vi "start ROI set-CCD1.vi"(0 "Rectangle big CCD1":T3 {"Rotation" format="%.2f"; "Left" scale=0.0..1024.0; "Right" scale=0.0..1024.0}, 1 "Rectangle small CCD1":T3 {"Rotation" format="%.2f"; "Left" scale=0.0..1024.0; "Right" scale=0.0..1024.0}, 2 "Line":T2 {"Start X" scale=0.0..1024.0; "End X" scale=0.0..1024.0}, 3 "Rectangle top CCD1":T3 {"Rotation" format="%.2f"; "Left" scale=0.0..1024.0; "Right" scale=0.0..1024.0}) -> (7 "ROI Descriptor (big)":T1={"Global Rectangle"=[1279, 916, 1775, 986], "Contours"=[{"ID"=enum."External", "Type"=12, "Coordinates"=[1280, 918, 1774, 984, 180289]}]} {"Contours"."Type" items=["No Selection", "Point", "Line", "Rectangle", "Oval", "Polygon", "Freehand Region", "Annulus", "Unused2", "Unused3", "Broken Line", "Freehand Line", "Rotated Rectangle"]}, 8 "ROI Descriptor (Small)":T1={"Global Rectangle"=[1279, 916, 1775, 986], "Contours"=[{"ID"=enum."External", "Type"=12, "Coordinates"=[1280, 918, 1774, 984, 180289]}]} {"Contours"."Type" items=["No Selection", "Point", "Line", "Rectangle", "Oval", "Polygon", "Freehand Region", "Annulus", "Unused2", "Unused3", "Broken Line", "Freehand Line", "Rotated Rectangle"]}, 9 "ROI Descriptor top":T1={"Global Rectangle"=[1279, 916, 1775, 986], "Contours"=[{"ID"=enum."External", "Type"=12, "Coordinates"=[1280, 918, 1774, 984, 180289]}]} {"Contours"."Type" items=["No Selection", "Point", "Line", "Rectangle", "Oval", "Polygon", "Freehand Region", "Annulus", "Unused2", "Unused3", "Broken Line", "Freehand Line", "Rotated Rectangle"]}, 10 "ROI Descriptor LINE":T1={"Global Rectangle"=[666, 165, 1207, 166], "Contours"=[{"ID"=enum."External", "Type"=2, "Coordinates"=[666, 165, 1206, 165]}]} {"Contours"."Type" items=["No Selection", "Point", "Line", "Rectangle", "Oval", "Polygon", "Freehand Region", "Annulus", "Unused2", "Unused3", "Broken Line", "Freehand Line", "Rotated Rectangle"]})   [LabVIEW 2017]
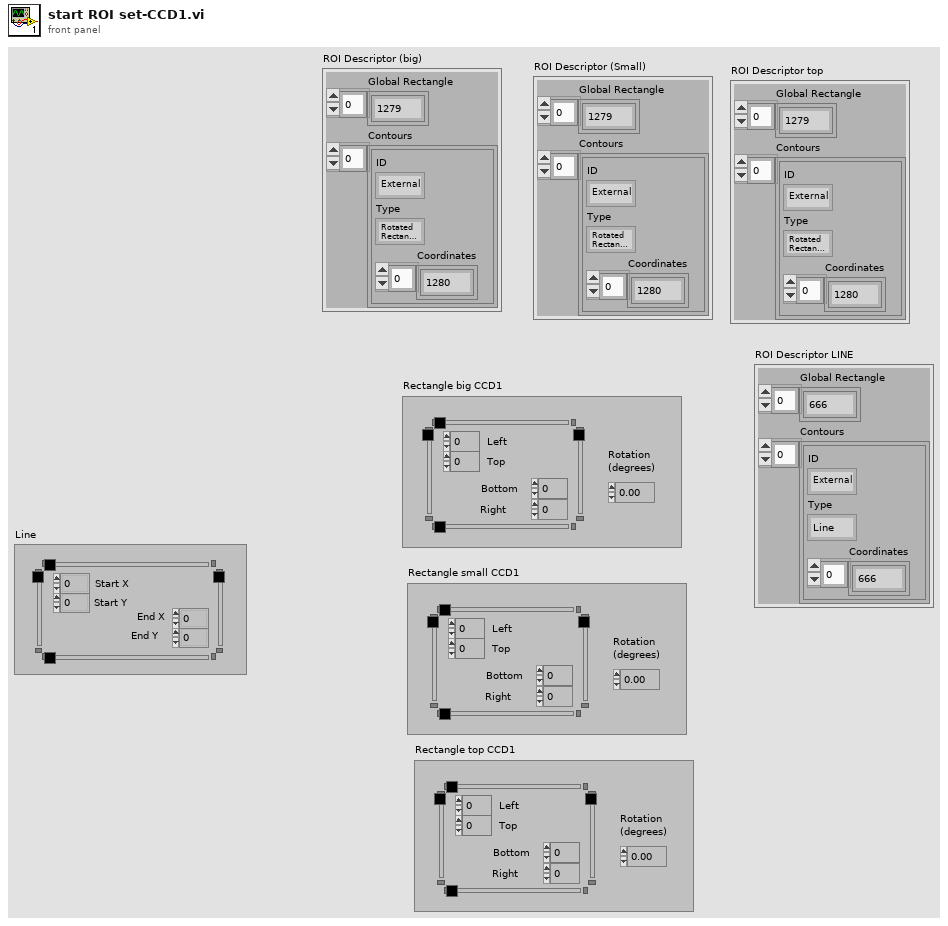
[diagram p1: front panel]
types:
  T1 = cluster{"Global Rectangle":i32[], "Contours":cluster{"ID":enum32{"External", "Internal"}, "Type":u32, "Coordinates":i32[]}[]}
  T2 = typedef "IMAQ Line" = cluster{"Start X":i32, "Start Y":i32, "End X":i32, "End Y":i32}
  T3 = typedef "IMAQ Rectangle" = cluster{"Left":i32, "Top":i32, "Right":i32, "Bottom":i32, "Rotation":dbl}
  T4 = typedef "ROI Descriptor" = cluster{"Global Rectangle":i32[], "Contours":cluster{"ID":enum32{"External", "Internal"}, "Type":u32, "Coordinates":i32[]}[]}
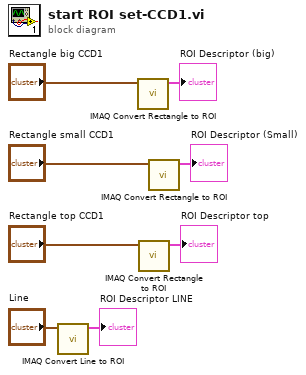
[diagram p0: block diagram]
diagram:
  n1 = call "IMAQ Convert Line to ROI"("Line"="Line") -> ("ROI Descriptor"=→"ROI Descriptor LINE":T4)  [unwired: 8 in, 1 out]
  n2 = call "IMAQ Convert Rectangle to ROI"("Rectangle"="Rectangle big CCD1") -> ("ROI Descriptor"=→"ROI Descriptor (big)":T4)  [unwired: 8 in, 1 out]
  n3 = call "IMAQ Convert Rectangle to ROI"("Rectangle"="Rectangle top CCD1") -> ("ROI Descriptor"=→"ROI Descriptor top":T4)  [unwired: 8 in, 1 out]
  n4 = call "IMAQ Convert Rectangle to ROI"("Rectangle"="Rectangle small CCD1") -> ("ROI Descriptor"=→"ROI Descriptor (Small)":T4)  [unwired: 8 in, 1 out]
